vi "lab2-2.vi"() -> ()   [LabVIEW 2014]
panel:
  out "Waveform Graph":dbl[](graph)
  out "scan freq":dbl
  in  "Stop Freq":dbl
  in  "Start Freq":dbl
  in  "Points":i32
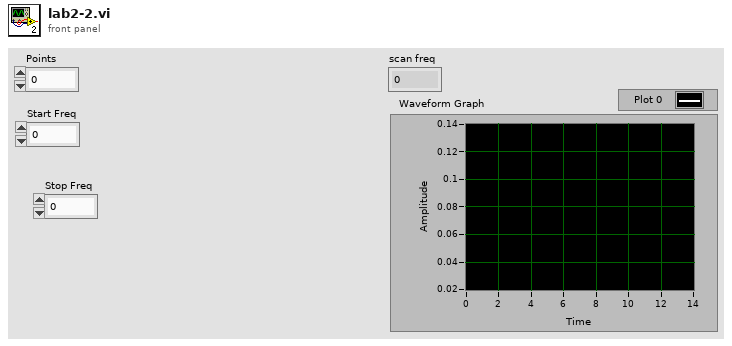
[diagram p1: front panel]
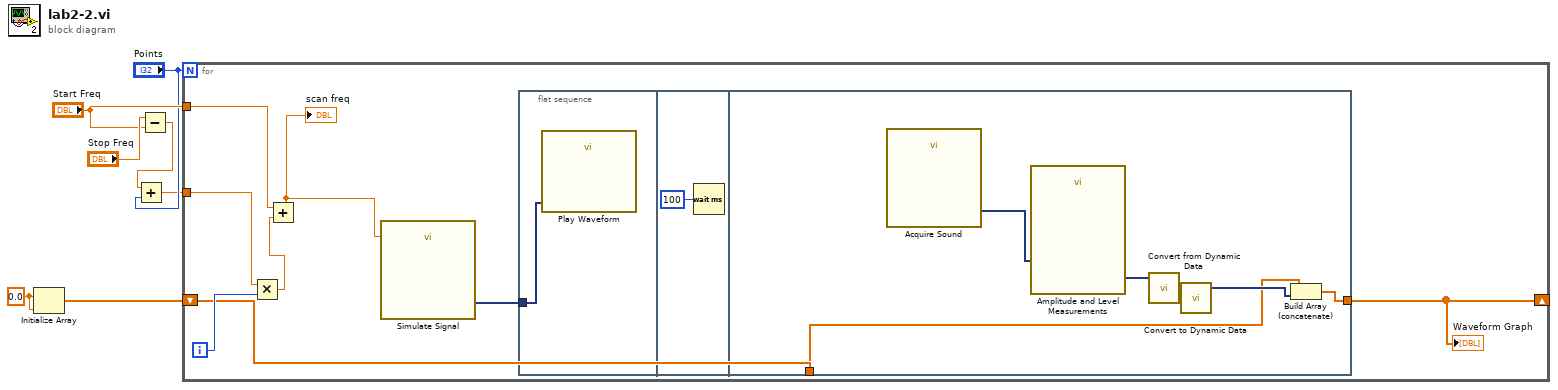
[diagram p0: block diagram]
diagram:
  w2 = 0.0 ("element")
  n1 = Initialize Array(w2, w2) -> (w1:dbl[])
  n2 = Subtract(x="Stop Freq", y="Start Freq") -> (x-y=w5:dbl)
  n3 = Add(x=w5, y="Points") -> (x+y=w3:dbl)
  n4 = for {
    N: "Points" -> [_]
    tunnel: "Start Freq" -> [w14]
    tunnel: w3 -> [w12]
    shift-right: [w8] -> _
    shift-left: w1 -> [w9]
    i -> [w15]
    n5 = Multiply(x=w12, y=w15) -> (x*y=w13:dbl)
    n6 = Add(x=w14, y=w13) -> (x+y=w10:dbl)
    "scan freq" <- w10
    n7 = call "Simulate Signal"("Frequency"=w10) -> ("Sine"=w11:dynamicdata)  [unwired: 13 in, 1 out]
    n8 = flat-sequence {
      tunnel: w11 -> [w16]
      tunnel: w9 -> [w19]
      tunnel: [w18] -> w8
      frame #0 {
        n9 = call "Play Waveform"("Data"=w16) -> ()  [unwired: 18 in, 1 out]
      }
      frame #1 {
        n10 = Wait (ms)(milliseconds to wait=u32 100) -> ()  [unwired: 1 out]
      }
      frame #2 {
        n11 = call "Acquire Sound"() -> ("Data"=w23:dynamicdata)  [unwired: 18 in, 1 out]
        n12 = call "Amplitude and Level Measurements"("Signals"=w23) -> ("Positive Peak"=w21:dynamicdata)  [unwired: 13 in, 1 out]
        n13 = call "Convert from Dynamic Data"("Dynamic Data Type"=w21) -> ("Array"=w20:dbl[])  [unwired: 3 in]
        n14 = call "Convert to Dynamic Data"("Array"=w20) -> ("Dynamic Data Type"=w22:dynamicdata)  [unwired: 3 in]
        n15 = Build Array (concatenate)(w19, w22) -> (w18:dbl[])
      }
    }
    "Waveform Graph" <- w8
  }
